vi "Read Temp UOM.vi"(8 "error in (no error)":errorcluster, 11 "Oven in":refnum<class "Oven.lvclass">) -> (0 "error out":errorcluster, 2 "Temp UOM":T1, 3 "Oven out":refnum<class "Oven.lvclass">)   [LabVIEW 2018, in "Oven.lvlib" / "Oven.lvclass"]
uses:
  Oven.lvclass
  Custom Controls/Temperature Unit of Measure.ctl
  Oven.lvclass/Oven.ctl
  Oven.lvlib
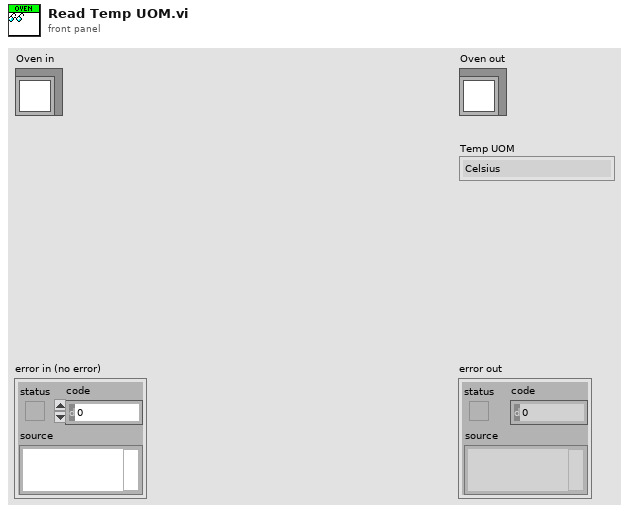
[diagram p1: front panel]
types:
  T1 = typedef "Oven.lvlib/Temperature Unit of Measure.ctl" = enum16{"Celsius", "Fahrenheit", "Kelvin"}
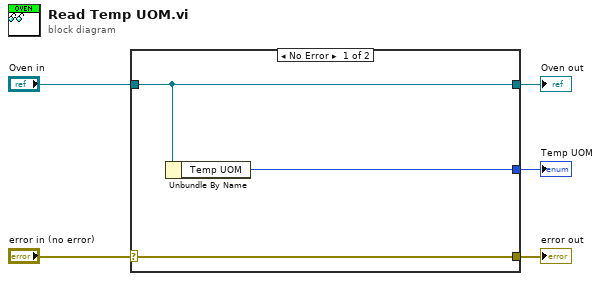
[diagram p0: block diagram]
diagram:
  n1 = case shown="No Error" "error in (no error)" {
    selector: "error in (no error)" -> [w8 w9]
    tunnel: [w8 w9] -> w4
    tunnel: [w7 w10] -> w2
    tunnel: "Oven in" -> [w7 w10]
    tunnel: [w6 _] -> w1
    frame No Error {
      n2 = Unbundle By Name(w7) -> ("Temp UOM"=w6:T1)
    }
    frame Error {
    }
  }
  "error out" <- w4
  "Oven out" <- w2
  "Temp UOM" <- w1
